vi "Custom XML Write.vi"(8 "error in (no error)":errorcluster, 9 "Prompt":string="Select Path to XML File", 10 "XML Input":string, 11 "XML File Path":path) -> (0 "error out":errorcluster, 2 "XML String":string, 3 "XML File Path(duplicate)":path)   [LabVIEW 2017]
doc: "Writes XML files without the <LVData> header."
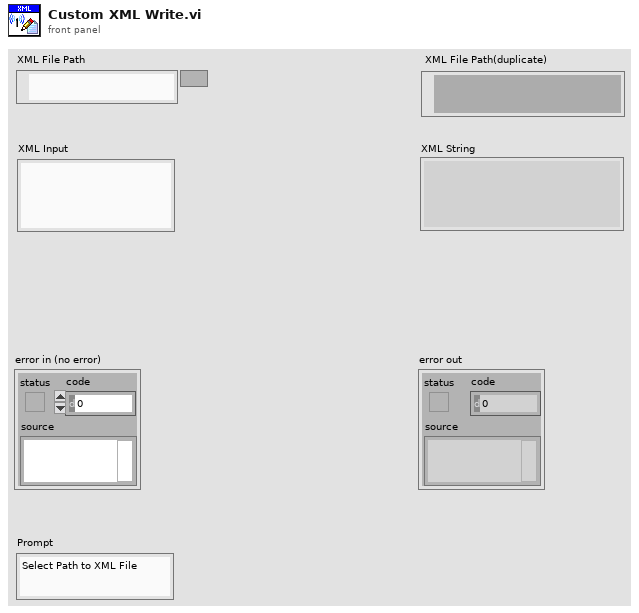
[diagram p1: front panel]
types:
  T1 = enum16{"open", "open or create", "create or replace", "create", "open (read only)"}
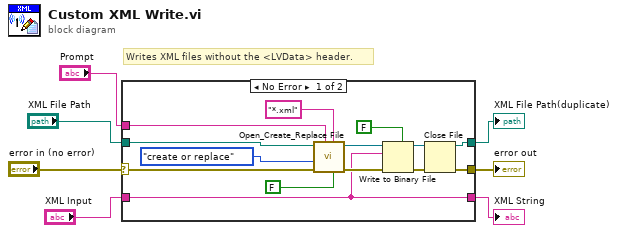
[diagram p0: block diagram]
diagram:
  # "Writes XML files without the <LVData> header."
  n1 = case shown="No Error" "error in (no error)" {
    selector: "error in (no error)" -> [w17 w24]
    tunnel: [w18 w24] -> w6
    tunnel: "XML Input" -> [w10 w23]
    tunnel: [w10 w23] -> w4
    tunnel: [w13 w22] -> w3
    tunnel: "XML File Path" -> [w9 w22]
    tunnel: "Prompt" -> [w8 _]
    frame No Error {
      n2 = call <vilib>:"Open_Create_Replace File.vi"("advisory dialog? (display:T)"=FALSE, "pattern"="*.xml", "prompt"=w8, "error in (no error)"=w17, "function (open:0)"=T1."create or replace", "file path"=w9) -> ("error out"=w20:errorcluster, "refnum"=w16:refnum<file>)  [unwired: 2 in, 2 out]
      n3 = Write to Binary File(file (use dialog)=w16, data=w10, error in=w20, 5:FALSE ("prepend array or string size? (T)")) -> (refnum out=w14:refnum<file>, error out=w19:errorcluster)  [unwired: 3 out]
      n4 = Close File(refnum=w14, error in=w19) -> (path=w13:path, error out=w18:errorcluster)
    }
    frame Error {
    }
  }
  "error out" <- w6
  "XML String" <- w4
  "XML File Path(duplicate)" <- w3
